vi "Actor Core.vi"(8 "error in":errorcluster, 11 "Nested in":refnum<class "UI.lvclass">) -> (0 "error out":errorcluster, 3 "Actor out":refnum<class "Actor.lvclass">)   [LabVIEW 2021, in "UI.lvlib" / "UI.lvclass"]
doc: "(<B>Filename</B>: Actor Framework.lvlib:Actor.lvclass:Actor Core.vi)\n\nReceives messages to the actor, reacts to them, and initiates any error handling that may shut the actor down.\n\nDescendant classes may override this VI to append parallel tasks for the actor to complete while it handles messages. Overrides use the Call Parent Method node."
uses:
  UI.lvclass
  C:/Program Files (x86)/National Instruments/LabVIEW 2021/vi.lib/ActorFramework/Actor/Actor.lvclass
  <vilib>/ActorFramework/Actor/Actor.lvclass
  Monedas/Monedas.lvclass
  Productos/Productos.lvclass
  UI.lvclass/UI.ctl
  Productos/Productos.lvclass/Productos.ctl
  Monedas/Monedas.lvclass/Monedas.ctl
  <vilib>/ActorFramework/Actor/Actor.lvclass/Actor.ctl
  <vilib>/ActorFramework/Message Enqueuer/Message Enqueuer.lvclass/Message Enqueuer.ctl
  <vilib>/ActorFramework/Message Enqueuer/Init from Existing Queue.vi
  <vilib>/ActorFramework/Message Enqueuer/Enqueue.vi
  <vilib>/ActorFramework/Stop Msg/Stop Msg.lvclass
  C:/Program Files (x86)/National Instruments/LabVIEW 2021/vi.lib/ActorFramework/Message/Message.lvclass
  <vilib>/ActorFramework/Message Priority Queue/Priority Enqueue.vi
  <vilib>/ActorFramework/Message Enqueuer/Message Enqueuer.lvclass
  C:/Users/scrap/Fork/Vending Machine AF/Actor-Framework-Vending-Machine/Vending Machine AF Folder/UI/UI.lvclass
  C:/Users/scrap/Fork/Vending Machine AF/Actor-Framework-Vending-Machine/Vending Machine AF Folder/Monedas/Monedas.lvclass
  C:/Users/scrap/Fork/Vending Machine AF/Actor-Framework-Vending-Machine/Vending Machine AF Folder/Productos/Productos.lvclass
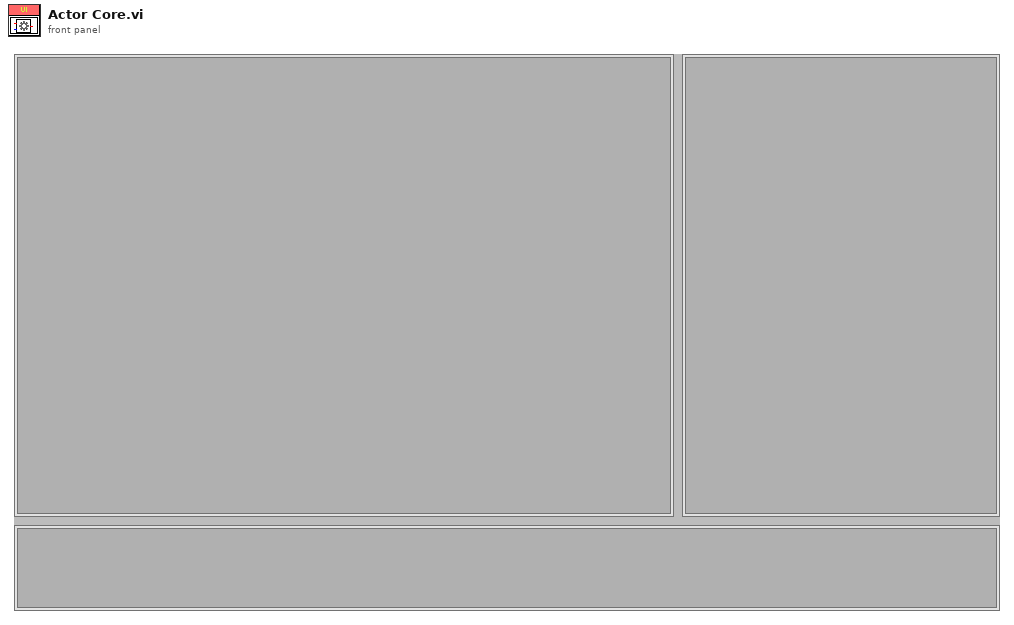
[diagram p1: front panel]
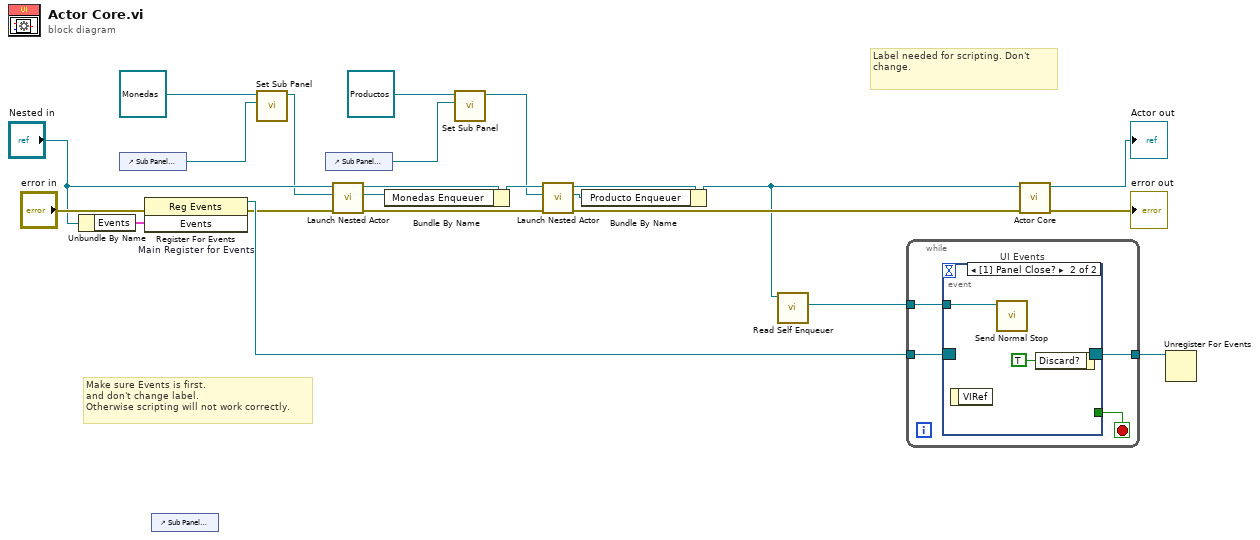
[diagram p0: block diagram]
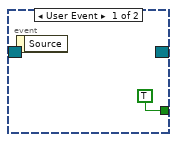
[diagram p2: hidden frame]
diagram:
  # "Label needed for scripting. Don't change."
  # "Make sure Events is first.\nand don't change label.\nOtherwise scripting will not work correctly."
  n1 = Unbundle By Name("Nested in") -> ("Events"=w20:cluster{"Stop":refnum<user-event>})
  n2 = control-ref of="Sub Panel Monedas"() -> (w13:refnum<vi>)
  n3 = register-events "Main Register for Events"(error in="error in", w20) -> (reference out=w21:refnum<event-registration>, error out=w16:errorcluster)  [unwired: 1 in]
  n4 = control-ref of="Sub Panel Mensajes"() -> ()  [unwired: 1 out]
  n5 = call "Set Sub Panel.vi"("Sub Panel"=w13, "Monedas in"=refnum<class "Monedas.lvclass"> refnum ("Monedas.lvlib:Monedas.lvclass")) -> ("Monedas out"=w12:refnum<class "Monedas.lvclass">)  [unwired: 8 in, 1 out]
  n6 = control-ref of="Sub Panel Proucto"() -> (w10:refnum<vi>)
  n7 = call <vilib>:"Launch Nested Actor.vi"("error in (no error)"=w16, "Nested Actor"=w12, "Caller Actor in"="Nested in") -> ("error out"=w7:errorcluster, "Nested Actor's Enqueuer"=w1:refnum<class "Message Enqueuer.lvclass">, "Caller Actor out"=w2:refnum<class "UI.lvclass">)  [unwired: 6 in]
  n8 = Bundle By Name(cluster=w2, "Monedas Enqueuer"=w1) -> (w9:refnum<class "UI.lvclass">)
  n9 = call "Set Sub Panel.vi"("Sub Panel"=w10, "Productos in"=refnum<class "Productos.lvclass"> refnum ("Productos.lvlib:Productos.lvclass")) -> ("Productos out"=w5:refnum<class "Productos.lvclass">)  [unwired: 8 in, 1 out]
  n10 = call <vilib>:"Launch Nested Actor.vi"("error in (no error)"=w7, "Nested Actor"=w5, "Caller Actor in"=w9) -> ("error out"=w6:errorcluster, "Nested Actor's Enqueuer"=w3:refnum<class "Message Enqueuer.lvclass">, "Caller Actor out"=w8:refnum<class "UI.lvclass">)  [unwired: 6 in]
  n11 = Bundle By Name(cluster=w8, "Producto Enqueuer"=w3) -> (w4:refnum<class "UI.lvclass">)
  n12 = call <vilib>:"Read Self Enqueuer.vi"("Actor"=w4) -> ("Self Enqueuer"=w18:refnum<class "Message Enqueuer.lvclass">)  [unwired: 10 in]
  n13 = while {
    tunnel: w21 -> [w27]
    tunnel: [w25] -> w19
    tunnel: w18 -> [w24]
    stop <- w26 stop-if-true
    n14 = event "UI Events" shown="[1] Panel Close?" {
      selector: w27 -> [_ _]
      dyn-events: [_ _] -> w25
      timeout: _ -> [_ _]
      tunnel: [TRUE _] -> w26
      tunnel: w24 -> [_ w29]
      event User Event {
        n15 = event-data() -> ()  [unwired: 1 in, 1 out]
      }
      event Panel Close? {
        n16 = event-data() -> ()  [unwired: 1 in, 1 out]
        n17 = call <vilib>:"Send Normal Stop.vi"("Message Enqueuer"=w29) -> ()  [unwired: 10 in, 1 out]
        n18 = event-data("Discard?"=TRUE) -> ()  [unwired: 1 in, 1 out]
      }
    }
  }
  n19 = call-parent "Actor Core.vi"("error in"=w6, "Actor in"=w4) -> ("error out"=→"error out":errorcluster, "Actor out"=→"Actor out":refnum<class "Actor.lvclass">)  [unwired: 8 in]
  n20 = Unregister For Events(event registration refnum=w19) -> ()  [unwired: 1 in, 1 out]
